vi "PLL analyzer -- publish -- async action.vi"(7 "publisher action":T2, 9 "asyncronous action":T1) -> (1 "asyncronous action OUT":T1)   [LabVIEW 2017]
uses:
  publisher action.ctl
  asyncronous action control.ctl
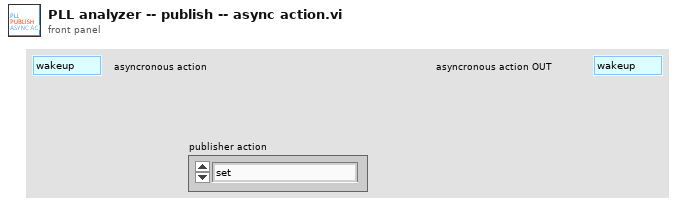
[diagram p1: front panel]
types:
  T1 = typedef "asyncronous action control.ctl" = enum16{"wakeup", "wait", "pause", "resume", "start", "stop"}
  T2 = typedef "publisher action.ctl" = enum16{"set", "get"}
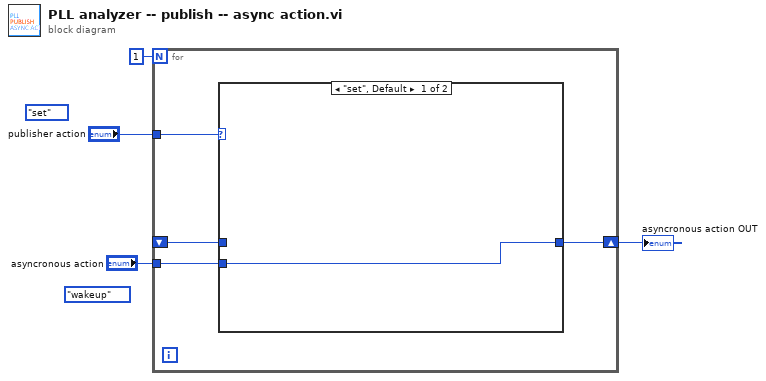
[diagram p0: block diagram]
diagram:
  (unwired) asyncronous_action_control."wakeup" ("asyncronous action")
  (unwired) publisher_action."set" ("publisher action")
  n1 = for {
    N: 1 -> [_]
    tunnel: "publisher action" -> [w8]
    shift-right: [w7] -> w1
    shift-left: _ -> [w5]
    tunnel: "asyncronous action" -> [w6]
    n2 = case shown="\"set\", Default" w8 {
      tunnel: [w9 w10] -> w7
      tunnel: w6 -> [w9 _]
      tunnel: w5 -> [_ w10]
      frame "set", Default {
      }
      frame "get" {
      }
    }
  }
  "asyncronous action OUT" <- w1
